vi "subExportOtherFileContent.vi"(6 "CodeSchema":string, 8 "error in (no error)":errorcluster, 9 "Expand?":bool, 10 "Add virtual folders?":bool, 11 "ILabVIEWItem in":refnum<class "ILabVIEWItem.lvclass">) -> (0 "error out":errorcluster, 1 "Links":T1, 2 "Nodes":T1, 3 "ILabVIEWItem out":refnum<class "ILabVIEWItem.lvclass">)   [LabVIEW 2020, in "DefaultExtensions.lvlib" / "CGrapherDGML.lvclass"]
uses:
  CGrapherDGML.lvclass
  obj/Addons/LabVIEWObjectInterfaces.lvlibp/LabVIEWObjectInterfaces/ILabVIEWItem/ILabVIEWItem.lvclass
  obj/Addons/LabVIEWItem.lvlibp/LabVIEWItem/CLabVIEWItem/ConnectionSet.ctl
  obj/Addons/LabVIEWItem.lvlibp/LabVIEWItem/CLabVIEWItem/CLabVIEWItem.lvclass
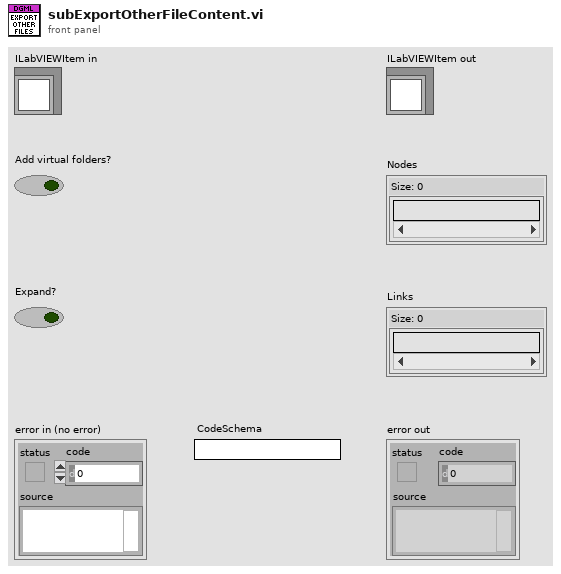
[diagram p1: front panel]
types:
  T1 = typedef "LabVIEWItem.lvlibp/CLabVIEWItem.lvclass/ConnectionSet.ctl" = set{string}
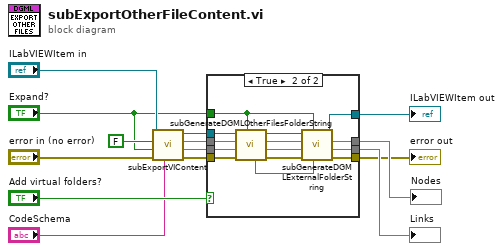
[diagram p0: block diagram]
diagram:
  n1 = call "subExportVIContent.vi"("CodeSchema"="CodeSchema", "error in (no error)"="error in (no error)", "Expand?"="Expand?", "Add virtual folders?"=FALSE, "ILabVIEWItem in"="ILabVIEWItem in") -> ("error out"=w10:errorcluster, "Links"=w12:T1, "Nodes"=w7:T1, "ILabVIEWItem out"=w9:refnum<class "ILabVIEWItem.lvclass">)  [unwired: 3 in]
  n2 = case shown="True" "Add virtual folders?" {
    tunnel: w12 -> [w15 w29]
    tunnel: [w15 w19] -> w11
    tunnel: w10 -> [w17 w31]
    tunnel: w9 -> [w18 w32]
    tunnel: [w18 w25] -> w8
    tunnel: w7 -> [w16 w30]
    tunnel: [w16 w20] -> w6
    tunnel: [w17 w27] -> w4
    tunnel: "Expand?" -> [_ w21]
    frame False {
    }
    frame True {
      n3 = call "subGenerateDGMLOtherFilesFolderString.vi"("Expand?"=w21, "error in (no error)"=w31, "Links in"=w29, "Nodes in"=w30, "ILabVIEWItem in"=w32) -> ("error out"=w28:errorcluster, "Links"=w23:T1, "Nodes"=w24:T1, "ILabVIEWItem out"=w26:refnum<class "ILabVIEWItem.lvclass">, "Path"=w22:string)  [unwired: 2 in]
      n4 = call "subGenerateDGMLExternalFolderString.vi"("Path in"=w22, "Expand?"=w21, "error in (no error)"=w28, "Links in"=w23, "Nodes in"=w24, "ILabVIEWItem in"=w26) -> ("error out"=w27:errorcluster, "Links"=w19:T1, "Nodes"=w20:T1, "ILabVIEWItem out"=w25:refnum<class "ILabVIEWItem.lvclass">)  [unwired: 2 in]
    }
  }
  "error out" <- w4
  "ILabVIEWItem out" <- w8
  "Nodes" <- w6
  "Links" <- w11
